vi "Build Driver Settings Mappings.vi"(8 "error in (no error)":errorcluster, 11 "DMM6500 in":refnum<class "DMM6500.lvclass">) -> (0 "error out":errorcluster, 3 "DMM6500 out":refnum<class "DMM6500.lvclass">)   [LabVIEW 2023, in "HAF.lvlib" / "DMM6500.lvclass"]
uses:
  DMM6500.lvclass
  DMM6500.lvclass/DMM6500.ctl
  Driver/Driver.lvclass
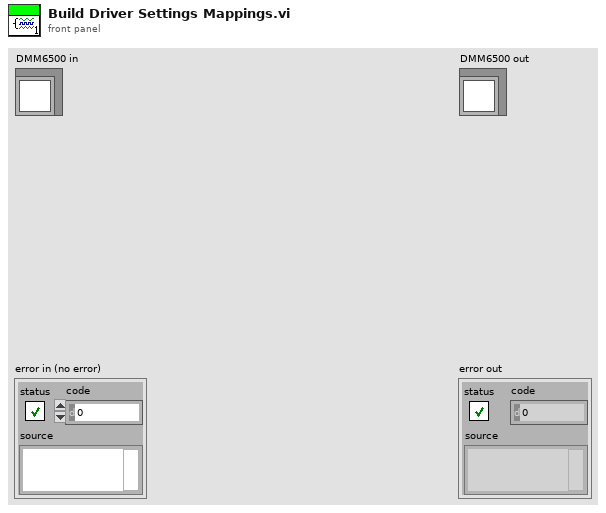
[diagram p1: front panel]
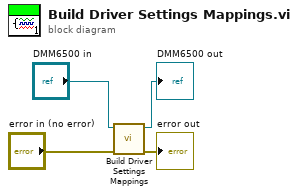
[diagram p0: block diagram]
diagram:
  n1 = call-parent "Build Driver Settings Mappings.vi"("error in (no error)"="error in (no error)", "Driver in"="DMM6500 in") -> ("error out"=→"error out":errorcluster, "Driver out"=→"DMM6500 out":refnum<class "DMM6500.lvclass">)  [unwired: 8 in]
